vi "BRig_dataCurrent_targetTPB.vi"() -> (2 "output_targetTPB":i32)   [LabVIEW 2014]
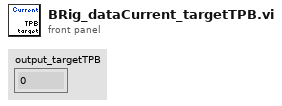
[diagram p1: front panel]
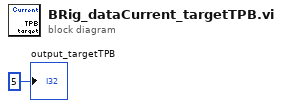
[diagram p0: block diagram]
diagram:
  "output_targetTPB" <- 5 ("output_iBlock")
